vi "ConfigAcq.vi"(8 "error in (no error)":errorcluster, 11 "Agilent_3458A in":refnum<class "Agilent_3458.lvclass">) -> (0 "error out":errorcluster, 3 "Agilent_3458A out":refnum<class "Agilent_3458.lvclass">)   [LabVIEW 2018, in "DigitizerPlugins.lvlib" / "Agilent_3458.lvclass"]
uses:
  Agilent_3458.lvclass
  C:/ICDAS/NistPluggableModules/Digitizer/DigitizerPlugins/DigitizerBaseClass/DigitizerBase.lvclass
  DigitizerBaseClass/DigitizerBase.lvclass/DigitizerBase.ctl
  Agilent_3458.lvclass/Agilent_3458.ctl
  DigitizerBaseClass/Accessors/Read InstRef.vi
  DigitizerBaseClass/Accessors/Read Acquisition.vi
  Accessors/Read Function (0_ DC Voltage).vi
  DigitizerBaseClass/Accessors/Read Channels.vi
  <instrlib>/Agilent 3458/Agilent 3458.lvlib
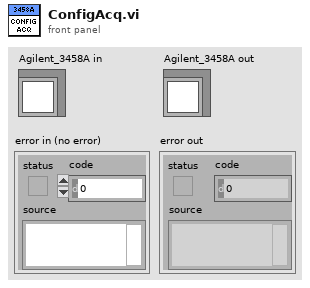
[diagram p1: front panel]
types:
  T1 = typedef "DigitizerPlugins.lvlib/DigitizerBase.lvclass/Acquisition.ctl" = cluster{"SampleRate":dbl, "RecordSize":i32, "NumRecords":i32, "SampleMode":i32, "Timeout (ms)":i32}
  T2 = typedef "DigitizerPlugins.lvlib/Agilent_3458.lvclass/MeasurementFunction.ctl" = i32
  T3 = typedef "DigitizerPlugins.lvlib/DigitizerBase.lvclass/Channel.ctl" = cluster{"Name":string, "Enabled":bool, "InputImpedance":dbl, "Coupling":enum16{"AC", "DC", "Gnd"}, "Offset":dbl, "Range":dbl}
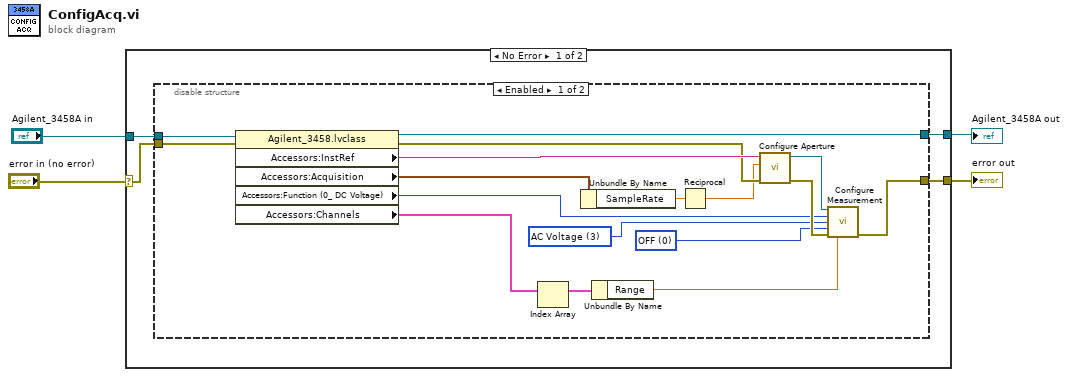
[diagram p0: block diagram]
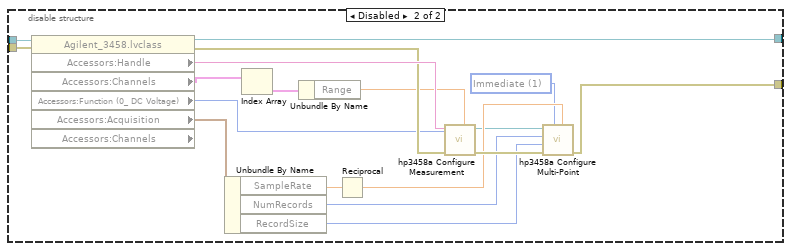
[diagram p2: hidden frame]
diagram:
  n1 = case shown="No Error" "error in (no error)" {
    selector: "error in (no error)" -> [w7 w45]
    tunnel: "Agilent_3458A in" -> [w8 w44]
    tunnel: [w6 w44] -> w2
    tunnel: [w5 w45] -> w1
    frame No Error {
      n2 = disable-structure shown="Enabled" {
        disable-tunnel: w8 -> [w25 w43]
        disable-tunnel: w7 -> [w24 w42]
        disable-tunnel: [w21 w31] -> w6
        disable-tunnel: [w16 w30] -> w5
        frame Enabled {
          w11 = u16 0 items=["OFF", "ON", "ONCE"] ("Auto Range (1:ON)")
          w14 = u16 3 items=["AC + DC Current", "AC + DC Voltage", "AC Current", "AC Voltage"] ("Frequency Source (3: AC Voltage)")
          n3 = property class="Agilent_3458.lvclass"(reference=w25, error in=w24) -> (reference out=w21:refnum<class "Agilent_3458.lvclass">, error out=w20:errorcluster, "Accessors:InstRef"=w23:string, "Accessors:Acquisition"=w22:T1, "Accessors:Function (0_ DC Voltage)"=w9:T2, "Accessors:Channels"=w10:T3[])
          n4 = Index Array(array=w10) -> (element=w13:T3)  [unwired: 1 in]
          n5 = Unbundle By Name(w22) -> ("SampleRate"=w19:dbl)
          n6 = Unbundle By Name(w13) -> ("Range"=w12:dbl)
          n7 = Reciprocal(x=w19) -> (1/x=w18:dbl)
          n8 = call <instrlib>:"Configure Aperture.vi"("error in (no error)"=w20, "Aperture Time (5.00E-9 s)"=w18, "VISA resource name"=w23) -> ("error out"=w17:errorcluster, "VISA resource name out"=w15:refnum<visa-resource-name>)  [unwired: 7 in]
          n9 = call <instrlib>:"Configure Measurement.vi"("VISA resource name"=w15, "Function (0: DC Voltage)"=w9, "Frequency Source (3: AC Voltage)"=w14, "Auto Range (1:ON)"=w11, "error in (no error)"=w17, "Manual Range (1.00)"=w12) -> ("error out"=w16:errorcluster)  [unwired: 8 in, 1 out]
        }
        frame Disabled {
          w32 = 1 items=["Immediate"=1, "External"=2, "Interval"=10, "Level"=1001, "Line"=1002] ("sample trigger (Immediate)")
          n10 = property class="Agilent_3458.lvclass" props=["Accessors:Handle", "Accessors:Channels", "Accessors:Function (0_ DC Voltage)", "Accessors:Acquisition", "Accessors:Channels"](reference=w43, error in=w42) -> (reference out=w31:refnum<class "Agilent_3458.lvclass">, error out=w40:errorcluster, "Accessors:Handle"=w41:string, "Accessors:Channels"=w39:T3[], "Accessors:Function (0_ DC Voltage)"=w29:T2, "Accessors:Acquisition"=w37:T1)  [unwired: 1 out]
          n11 = Unbundle By Name(w37) -> ("SampleRate"=w35:dbl, "NumRecords"=w27:i32, "RecordSize"=w26:i32)
          n12 = Index Array(array=w39) -> (element=w38:T3)  [unwired: 1 in]
          n13 = Unbundle By Name(w38) -> ("Range"=w28:dbl)
          n14 = Reciprocal(x=w35) -> (1/x=w34:dbl)
          n15 = call <instrlib>:"hp3458a Configure Measurement.vi"("range (-1:Auto)"=w28, "error in (no error)"=w40, "measurement function (DC V)"=w29, "instrument handle"=w41) -> ("error out"=w36:errorcluster, "instrument handle out"=w33:refnum<k15>)  [unwired: 6 in]
          n16 = call <instrlib>:"hp3458a Configure Multi-Point.vi"("sample interval (1.00E+0 s)"=w34, "sample trigger (Immediate)"=w32, "error in (no error)"=w36, "sample count (1)"=w26, "trigger count (1)"=w27, "instrument handle"=w33) -> ("error out"=w30:errorcluster)  [unwired: 4 in, 1 out]
        }
      }
    }
    frame Error {
    }
  }
  "error out" <- w1
  "Agilent_3458A out" <- w2
